vi "Spawn Child placeholder.vi"(11 "TEMPLATE Actor in":refnum<class "{{Name}}Actor.lvclass">) -> (0 "Error out":errorcluster, 3 "TEMPLATE Actor out":refnum<class "{{Name}}Actor.lvclass">)   [LabVIEW 2020, in "_Template.lvlib" / "Templates.lvlib" / "{{Name}}Actor.lvlib" / "{{Name}}Actor.lvclass"]
uses:
  {{Name}}Actor.lvclass
  {{Name}}Actor.lvclass/{{Name}}Actor.ctl
  jettl/jettl/Actor/Actor.lvclass
  Child Aliases.ctl
  jettl/jettl/jettl.lvlib
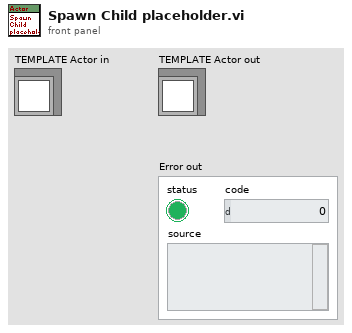
[diagram p1: front panel]
types:
  T1 = typedef "_Template.lvlib/Templates.lvlib/{{Name}}Actor.lvlib/{{Name}}Actor.lvclass/Child Aliases.ctl" = enum16{"placeholder"}
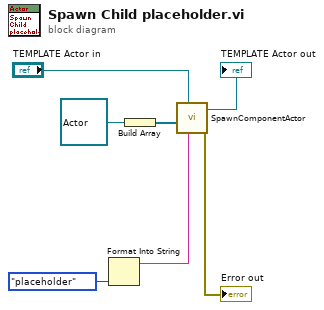
[diagram p0: block diagram]
diagram:
  n1 = Format Into String(Child_Aliases."placeholder" ("Child UIDs")) -> (resulting string=w2:string)  [unwired: 3 in, 1 out]
  n2 = Build Array(refnum<class "Actor.lvclass"> refnum ("Actor")) -> (w5:refnum<class "Actor.lvclass">[])
  n3 = call "SpawnComponentActor.vi"("Unified Actor Alias"=w2, "Actor in"="TEMPLATE Actor in", "Actors"=w5) -> ("Error out"=→"Error out":errorcluster, "Actor out"=→"TEMPLATE Actor out":refnum<class "Actor.lvclass">)  [unwired: 7 in]
